vi "convert_double_to_string.vi"(4 "double in":dbl format="%#.12g", 5 "String to add before (\"\")":string) -> (1 "string out":string)   [LabVIEW 2014, in "rszvl_rsidr_core.lvlib"]
uses:
  rszvl_rsidr_core.lvlib
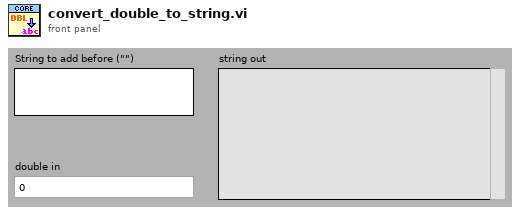
[diagram p1: front panel]
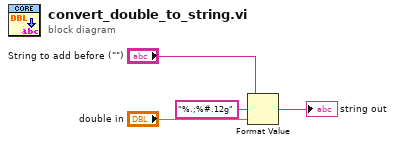
[diagram p0: block diagram]
diagram:
  n1 = Format Value(string ("")="String to add before (\"\")", format string="%.;%#.12g", value (0)="double in") -> (output string=→"string out":string)
